vi "Simple Move.vi"() -> ()   [LabVIEW 2023]
doc: "Demonstrates the Move method in VI Scripting to programmatically move an object from one location to another, where the destination is a block diagram."
uses:
  <vilib>/Utility/miscctls.llb/LVPositionTypeDef.ctl
panel:
  in  "Add Label":string="Move Me - Add"
  # "Overview: Demonstrates the Move method in VI Scripting to programmatically move an object from one location to another.\nInstructions:\n1. Open the block diagrams of Test - Moving Objects Source.vi and Test - Moving Objects Target.vi.\n2. Run this VI. The \"Move Me - Add\" function will be copied from the source VI into the target VI.\n\nNote: When moving an object from one VI to another, the operation results in a copy, since the original object is preserved. When moving an object to a different location in the same VI, it will not be a copy operation unless the Duplicate? parameter of the Move method is set to TRUE."
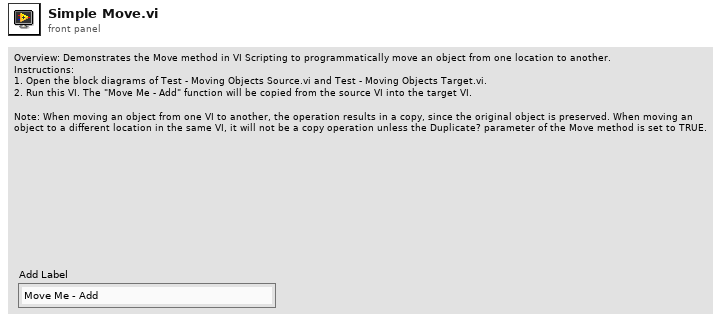
[diagram p1: front panel]
types:
  T1 = typedef "LVPositionTypeDef.ctl" = cluster{"Left":i32, "Top":i32}
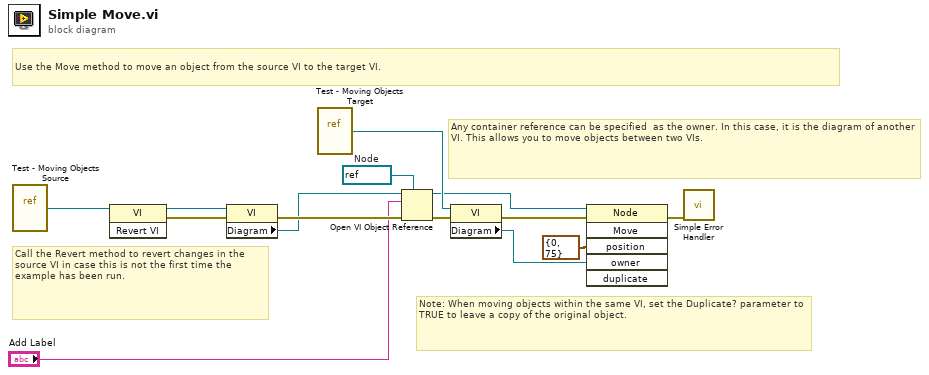
[diagram p0: block diagram]
diagram:
  w5 = refnum<vi> refnum  # Node
  # "Use the Move method to move an object from the source VI to the target VI."
  # "Note: When moving objects within the same VI, set the Duplicate? parameter to TRUE to leave a copy of the original object."
  # "Any container reference can be specified  as the owner. In this case, it is the diagram of another VI. This allows you to move objects between two VIs."
  # "Call the Revert method to revert changes in the source VI in case this is not the first time the example has been run."
  n1 = vi-ref "Test - Moving Objects Source.vi"() -> (w13:refnum<vi>)
  n2 = invoke class="VI" method="Revert VI"(reference=w13) -> (reference out=w12:refnum<vi>, error out=w11:errorcluster)  [unwired: 2 in, 1 out]
  n3 = property class="VI"(reference=w12, error in=w11) -> (error out=w8:errorcluster, "Diagram"=w2:refnum<vi>)  [unwired: 1 out]
  n4 = vi-ref "Test - Moving Objects Target.vi"() -> (w14:refnum<vi>)
  n5 = Open VI Object Reference(7:w5, 8:w8, 10:"Add Label", 11:w2) -> (0:w7:errorcluster, 3:w9:refnum<vi>)
  n6 = property class="VI"(reference=w14, error in=w7) -> (error out=w6:errorcluster, "Diagram"=w1:refnum<vi>)  [unwired: 1 out]
  n7 = invoke class="Node" method="Move"(reference=w9, error in=w6, "position"=T1 {"Left"=0, "Top"=75}, "owner"=w1) -> (error out=w10:errorcluster)  [unwired: 2 in, 5 out]
  n8 = call <vilib>:"Simple Error Handler.vi"("error in (no error)"=w10) -> ()  [unwired: 4 in, 5 out]
